vi "sendCmd.vi"(3 "error in":errorcluster, 4 "Command":string="sRN LMDscandata", 5 "connection ID":refnum<k5>) -> (0 "error out":errorcluster, 1 "Response":string, 2 "connection ID":refnum<k5>)   [LabVIEW 2009]
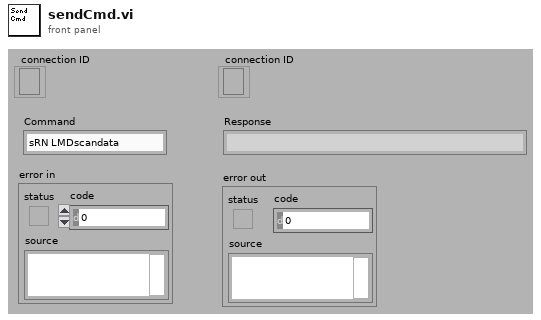
[diagram p1: front panel]
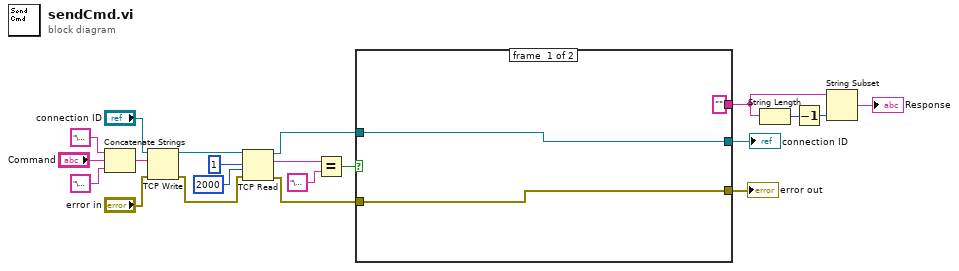
[diagram p0: block diagram]
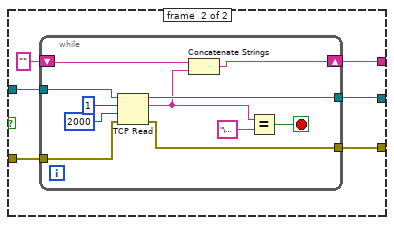
[diagram p2: hidden frame]
diagram:
  n1 = Concatenate Strings("\u0002" ("string"), "Command", "\u0003" ("string")) -> (w5:string)
  n2 = TCP Write(connection ID="connection ID", data in=w5, error in (no error)="error in") -> (connection ID out=w6:refnum<k5>, error out=w8:errorcluster)  [unwired: 1 in, 1 out]
  n3 = TCP Read(connection ID=w6, bytes to read=1, error in (no error)=w8, 9:2000 ("timeout ms (25000)")) -> (connection ID out=w18:refnum<k5>, data out=w14:string, error out=w19:errorcluster)  [unwired: 1 in]
  n4 = Equal?(x=w14, y="\u0002") -> (x = y?=w17:bool)
  n5 = case shown="True" w17 {
    tunnel: w18 -> [w23 w30]
    tunnel: w19 -> [w22 w29]
    tunnel: ["" w27] -> w3
    tunnel: [w23 w26] -> w20
    tunnel: [w22 w25] -> w21
    frame #0 {
    }
    frame #1 {
      n6 = while {
        tunnel: w30 -> [w40]
        tunnel: w29 -> [w39]
        shift-right: [w38] -> w27
        shift-left: "" -> [w37]
        tunnel: [w36] -> w26
        tunnel: [w33] -> w25
        stop <- w34 stop-if-true
        n7 = TCP Read(connection ID=w40, bytes to read=1, error in (no error)=w39, 9:2000 ("timeout ms (25000)")) -> (connection ID out=w36:refnum<k5>, data out=w32:string, error out=w33:errorcluster)  [unwired: 1 in]
        n8 = Concatenate Strings(w37, w32) -> (w38:string)
        n9 = Equal?(x=w32, y="\u0003") -> (x = y?=w34:bool)
      }
    }
  }
  "connection ID" <- w20
  "error out" <- w21
  n10 = String Length(string=w3) -> (length=w2:i32)
  n11 = Decrement(x=w2) -> (x-1=w1:i32)
  n12 = String Subset(string=w3, length (rest)=w1) -> (substring=→"Response":string)  [unwired: 1 in]
